vi "Get ClassName.vi"(8 "error in (no error)":errorcluster, 11 "Message in":refnum<class "Message.lvclass">) -> (0 "error out":errorcluster, 2 "Class Name":string, 3 "Message out":refnum<class "Message.lvclass">)   [LabVIEW 2009, in "LapDog.Messaging.v2.lvlib" / "Message.lvclass"]
doc: "Returns the <b>class name</b> (not message name) of the object on the wire at runtime. Class Name does not return the fully qualified name of the object nor the .lvclass extension.\n\nThis method executes regardless of the error in state."
uses:
  Message.lvclass
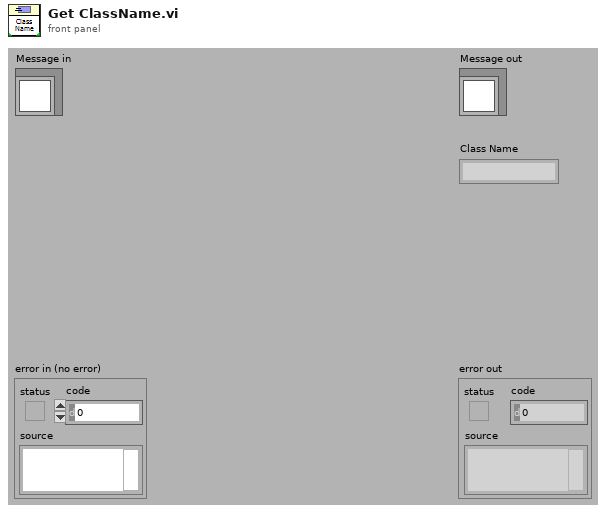
[diagram p1: front panel]
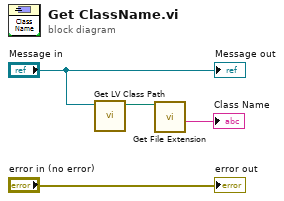
[diagram p0: block diagram]
diagram:
  n1 = call <vilib>:"Get LV Class Path.vi"("object"="Message in") -> ("class path"=w1:path)  [unwired: 1 in, 9 out]
  n2 = call <vilib>:"Get File Extension.vi"("file"=w1) -> ("filename without extension"=→"Class Name":string)  [unwired: 1 in, 9 out]
  "error out" <- "error in (no error)"
  "Message out" <- "Message in"
